vi "Append Report Text (num).vi"(0 "report in":refnum<class "ooCalc.lvclass">, 1 "MS Office parameters":T1, 2 "format string (%.3f)":string="%.3f", 7 "text":dbl format="%.2f", 9 "append on new line? (F)":bool, 11 "error in (no error)":errorcluster) -> (4 "report out":refnum<class "ooCalc.lvclass">, 8 "start out (Word)":i32, 10 "end out (Word)":i32, 15 "error out":errorcluster)   [LabVIEW 2009, in "ooCalc.lvclass"]
doc: "Appends text to the selected report."
uses:
  ooCalc.lvclass
  <vilib>/Utility/NIReport.llb/Append Report Text (str wrap).vi
  <vilib>/Utility/NIReport.llb/NI_report.lvclass
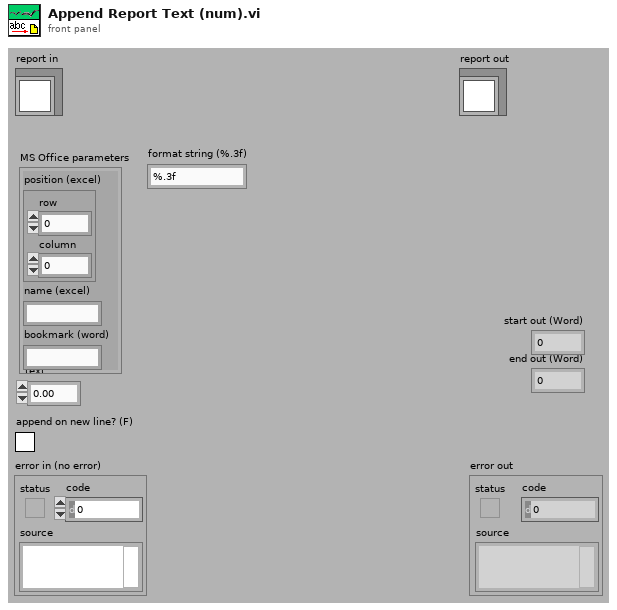
[diagram p1: front panel]
types:
  T1 = cluster{"position (excel)":cluster{"row":i32, "column":i32}, "name (excel)":string, "bookmark (word)":string}
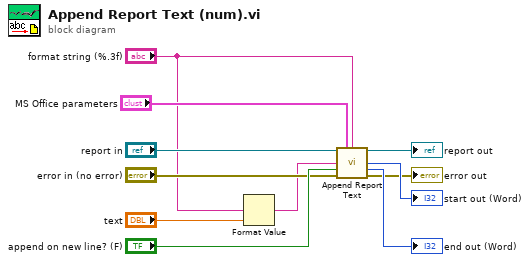
[diagram p0: block diagram]
diagram:
  n1 = Format Value(format string="format string (%.3f)", value (0)="text") -> (output string=w1:string)  [unwired: 1 in]
  n2 = call-poly <vilib>:"Append Report Text.vi"("report in"="report in", "MS Office parameters"="MS Office parameters", "format string (%.3f)"="format string (%.3f)", "text"=w1, "append on new line? (F)"="append on new line? (F)", "error in (no error)"="error in (no error)") -> ("report out"=→"report out":refnum<class "ooCalc.lvclass">, "start out (Word)"=→"start out (Word)":i32, "end out (Word)"=→"end out (Word)":i32, "error out"=→"error out":errorcluster)  [unwired: 6 in]
